vi "Set discriminator scan step size.vi"(8 "error in (no error)":errorcluster, 9 "v (0.000000)":dbl, 10 "i (0)":T1, 11 "VISA resource name":refnum<visa-resource-name>) -> (0 "error out":errorcluster, 3 "VISA resource name out":refnum<visa-resource-name>)   [LabVIEW 2009, in "SR400.lvlib"]
doc: "DY i { ,v }\nThe DY command sets and reads the discriminator\nscan step size. i = 0,1, or 2 designates\ndiscriminator A,B, or T and is required. If v is\nincluded, the selected discriminator scan step is set\nto v Volts where -0.0200 <= v <= 0.0200. The\nresolution is 0.0002 V (0.2 mV). If v is absent, the\nselected discriminator scan step is returned. The\nscan step may be set and read even if the selected discriminator is in the FIXED mode. Changing the\nscan step during a scan will affect the level for the\nnext count period and all those that follow."
uses:
  SR400.lvlib
  Typedefs.llb/Counter.ctl
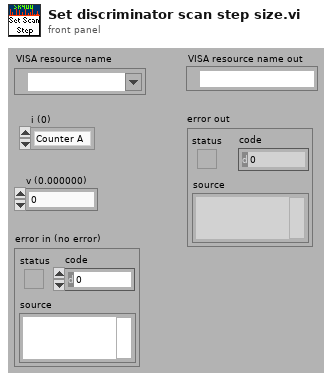
[diagram p1: front panel]
types:
  T1 = typedef "SR400.lvlib/Counter.ctl" = enum16{"Counter A", "Counter B", "Counter T"}
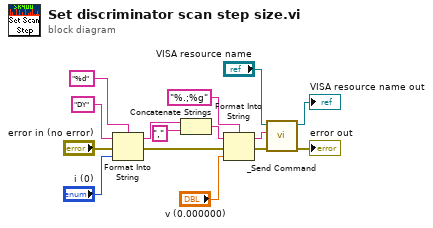
[diagram p0: block diagram]
diagram:
  n1 = Format Into String(format string="%d", initial string="DY" ("command"), error in="error in (no error)", "i (0)") -> (resulting string=w12:string, error out=w13:errorcluster)
  n2 = Concatenate Strings(w12, "," ("command")) -> (w7:string)
  n3 = Format Into String(format string="%.;%g", initial string=w7, error in=w13, "v (0.000000)") -> (resulting string=w4:string, error out=w3:errorcluster)
  n4 = call "_Send Command.vi"("error in (no error)"=w3, "Command"=w4, "VISA resource name"="VISA resource name") -> ("error out"=→"error out":errorcluster, "VISA resource name out"=→"VISA resource name out":refnum<visa-resource-name>)  [unwired: 1 in, 6 out]
